vi "Delete ROI.vi"(8 "error in (no error)":errorcluster, 11 "IMAQ Display in":refnum<class "HIJ Vision Display.lvclass">) -> (0 "error out":errorcluster, 3 "IMAQ Display out":refnum<class "HIJ Vision Display.lvclass">)   [LabVIEW 2014, in "HIJ Vision Display.lvlib" / "HIJ Vision Display.lvclass"]
uses:
  HIJ Vision Display.lvclass
  HIJ Vision Display.lvclass/HIJ Vision Display.ctl
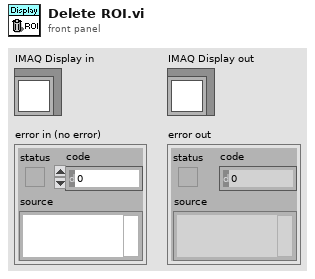
[diagram p1: front panel]
types:
  T1 = typedef "HIJ Vision Display.lvlib/HIJ Vision Display.lvclass/Named ROI.ctl" = cluster{"ROI":cluster{"Global Rectangle":i32[], "Contours":cluster{"Contour Type":u32, "ROI Type":u32, "Points":i32[]}[]}, "Name":string}
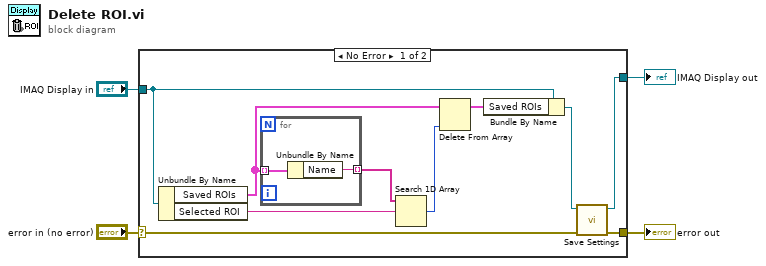
[diagram p0: block diagram]
diagram:
  n1 = case shown="No Error" "error in (no error)" {
    selector: "error in (no error)" -> [w6 w18]
    tunnel: [w5 w18] -> w3
    tunnel: [w7 w17] -> w1
    tunnel: "IMAQ Display in" -> [w9 w17]
    frame No Error {
      n2 = Unbundle By Name(w9) -> ("Saved ROIs"=w12:T1[], "Selected ROI"=w10:string)
      n3 = for {
        tunnel: w12 -> [w16] mode=indexing
        tunnel: [w15] -> w11 mode=indexing
        n4 = Unbundle By Name(w16) -> ("Name"=w15:string)
      }
      n5 = Search 1D Array(1D array=w11, element=w10) -> (index of element=w13:i32)  [unwired: 1 in]
      n6 = Delete From Array(array=w12, index=w13) -> (array with subset deleted=w14:T1[])  [unwired: 1 in, 1 out]
      n7 = Bundle By Name(cluster=w9, "Saved ROIs"=w14) -> (w8:refnum<class "HIJ Vision Display.lvclass">)
      n8 = call-dynamic "Save Settings.vi"("error in (no error)"=w6, "IMAQ Display in"=w8) -> ("error out"=w5:errorcluster, "IMAQ Display out"=w7:refnum<class "HIJ Vision Display.lvclass">)  [unwired: 8 in]
    }
    frame Error {
    }
  }
  "error out" <- w3
  "IMAQ Display out" <- w1
